vi "APS pt get error.vi"(8 "error in (no error)":errorcluster caption="错误输入（无错误）", 9 "ErrCode":i32, 10 "PtbId":i32, 11 "Board_ID":i32) -> (0 "error out":errorcluster caption="错误输出", 1 "ErrCode out":i32, 3 "function return":i32)   [LabVIEW 2011, in "APS168.lvlib"]
doc: "I32 FNTYPE APS_pt_get_error( I32 Board_ID, I32 PtbId, I32 *ErrCode );"
uses:
  APS168.lvlib
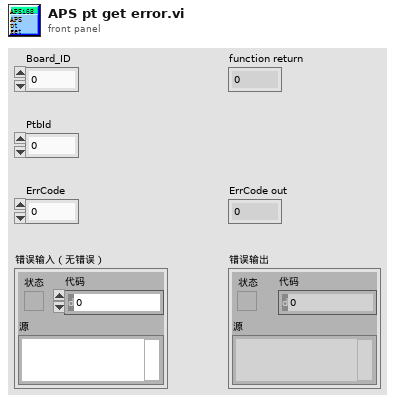
[diagram p1: front panel]
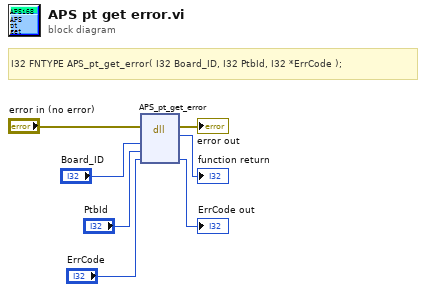
[diagram p0: block diagram]
diagram:
  # "I32 FNTYPE APS_pt_get_error( I32 Board_ID, I32 PtbId, I32 *ErrCode );"
  n1 = dll-call lib="PTH1Labs E软件ADLINK 204CAPS_1_7_1_LIB line 连续运动204APS168.*" fn="APS_pt_get_error"(error in="error in (no error)", "Board_ID"="Board_ID", "PtbId"="PtbId", "ErrCode"="ErrCode") -> (error out=→"error out":errorcluster, →"function return":i32, "ErrCode"=→"ErrCode out":i32)  [unwired: 4 in, 1 out]
